vi "Auto_Flywheel_Speed_Control.vi"() -> (1 "RPM output":dbl)   [LabVIEW 2019]
uses:
  Globals/Sensor_Values.vi
panel:
  out "subarray":dbl[](array[numeric])
  out "Array Index":dbl
  out "Fractional Index":dbl
  out "Search Value":dbl
  out "Input File":string
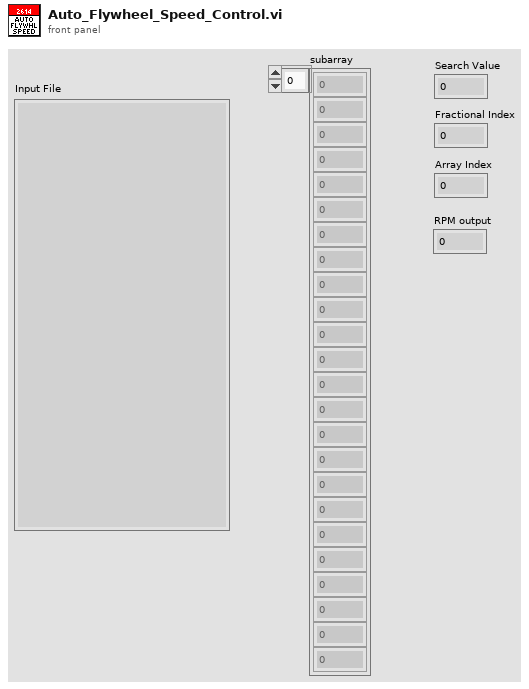
[diagram p1: front panel]
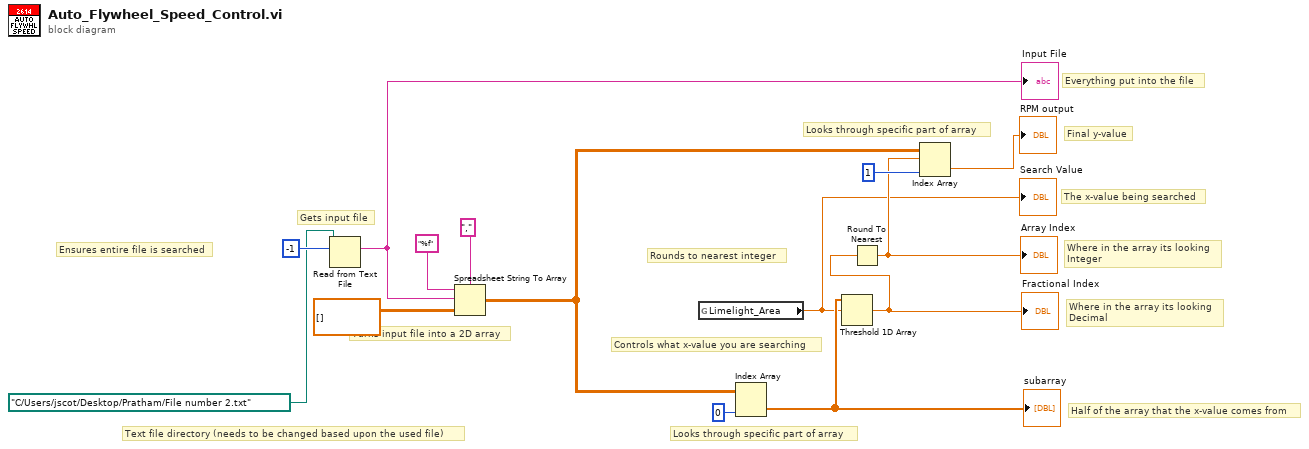
[diagram p0: block diagram]
diagram:
  # "Ensures entire file is searched"
  # "Looks through specific part of array"
  # "Looks through specific part of array"
  # "Half of the array that the x-value comes from"
  # "Gets input file"
  # "Turns input file into a 2D array"
  # "Rounds to nearest integer"
  # "Controls what x-value you are searching"
  # "Everything put into the file"
  # "The x-value being searched"
  # "Where in the array its looking\nInteger"
  # "Where in the array its looking\nDecimal"
  # "Final y-value"
  # "Text file directory (needs to be changed based upon the used file)"
  n1 = Read from Text File(file (use dialog)=path "C:/Users/jscot/Desktop/Pratham/File number 2.txt", count=-1) -> (text=w9:string)  [unwired: 2 in, 3 out]
  "Input File" <- w9
  n2 = Spreadsheet String To Array(delimiter (Tab)=",", format string="%f", spreadsheet string=w9, array type (2D Dbl)=dbl[][] []) -> (array=w5:dbl[][])
  n3 = global read "Sensor_Values.vi" "Limelight_Area"() -> (w1:dbl)
  "Search Value" <- w1
  n4 = Index Array(array=w5, index (col)=0 ("disabled index (col)")) -> (element=w7:dbl[])  [unwired: 1 in]
  "subarray" <- w7
  n5 = Threshold 1D Array(2:w1, 3:w7) -> (0:w6:dbl)  [unwired: 1 in]
  "Fractional Index" <- w6
  n6 = Round To Nearest(number=w6) -> (nearest integer value=w2:dbl)
  "Array Index" <- w2
  n7 = Index Array(array=w5, index (row)=w2, index (col)=1 ("disabled index (row)")) -> (element=→"RPM output":dbl)
